vi "Configure.vi"(8 "error in":errorcluster, 11 "File Actor in":refnum<class "File Actor.lvclass">) -> (0 "error out":errorcluster, 3 "File Actor out":refnum<class "File Actor.lvclass">)   [LabVIEW 2016, in "File Library.lvlib" / "File Actor.lvclass"]
uses:
  File Actor.lvclass
  C:/Program Files (x86)/National Instruments/LabVIEW 2016/vi.lib/ActorFramework/Actor/Actor.lvclass
  C:/Program Files (x86)/National Instruments/LabVIEW 2016/vi.lib/MSR Consulting, LLC/General Reuse/SuperActor/SuperActor.lvclass
  <vilib>/MSR Consulting, LLC/General Reuse/Session APIs/File Access/Config Data/Config Data.lvclass
  Messages/To/Save/Change File Writing State MSG.lvclass
  C:/Program Files (x86)/National Instruments/LabVIEW 2016/vi.lib/ActorFramework/Message/Message.lvclass
  <vilib>/ActorFramework/Actor/Actor.lvclass/Actor.ctl
  <vilib>/ActorFramework/Message Enqueuer/Message Enqueuer.lvclass/Message Enqueuer.ctl
  File Actor.lvclass/File Actor.ctl
  <vilib>/MSR Consulting, LLC/General Reuse/SuperActor/SuperActor.lvclass/SuperActor.ctl
  <vilib>/MSR Consulting, LLC/General Reuse/Session APIs/File Access/Config Data/Config Data.lvclass/Config Data.ctl
  Messages/To/Save/Change File Writing State MSG.lvclass/Change File Writing State MSG.ctl
  Read Cfg Header.vi
  <vilib>/MSR Consulting, LLC/General Reuse/SuperActor/Read ID.vi
  <vilib>/MSR Consulting, LLC/General Reuse/SuperActor/Read Config Session.vi
  <vilib>/MSR Consulting, LLC/General Reuse/Session APIs/File Access/Config Data/Accessors/Read Ref.vi
  Messages/To/Save/Write Save_.vi
  <vilib>/ActorFramework/Message Enqueuer/Init from Existing Queue.vi
  <vilib>/Utility/config.llb/Read Key (String).vi
  <vilib>/Utility/config.llb/Read Key (Boolean).vi
  <vilib>/Utility/config.llb/Read Key (I32).vi
  <vilib>/ActorFramework/Message Priority Queue/Priority Enqueue.vi
  <vilib>/ActorFramework/Message Enqueuer/Message Enqueuer.lvclass
  <vilib>/MSR Consulting, LLC/General Reuse/Session APIs/_Session Fwk/Session - Root.lvclass
  <vilib>/Utility/config.llb/NI_LVConfig.lvlib
  <vilib>/ActorFramework/Actor/Actor.lvclass
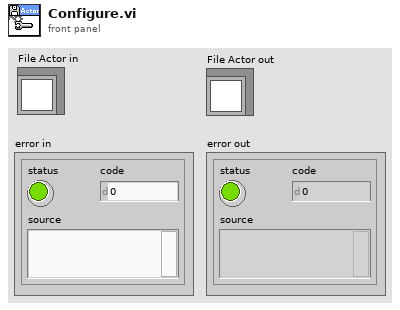
[diagram p1: front panel]
types:
  T1 = typedef "Session - Root.lvclass/Session Handle.ctl" = refnum<data-value>
  T2 = typedef "NI_LVConfig.lvlib/Config Data RefNum.ctl" = refnum<k1>
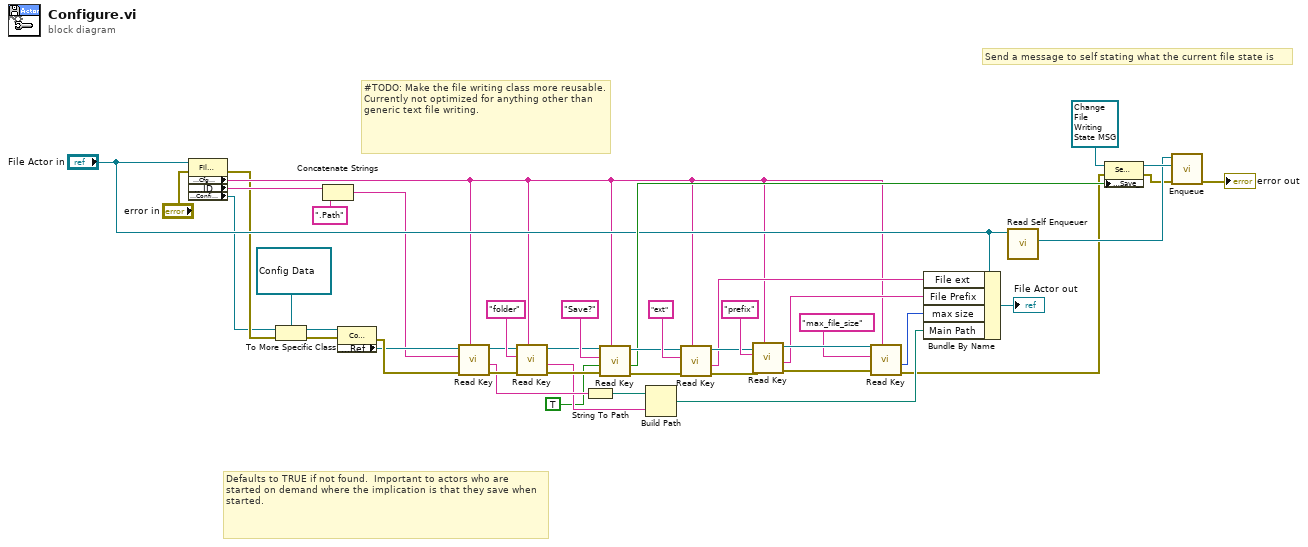
[diagram p0: block diagram]
diagram:
  # "Defaults to TRUE if not found.  Important to actors who are started on demand where the implication is that they save when started."
  # "Send a message to self stating what the current file state is"
  # "#TODO: Make the file writing class more reusable.  Currently not optimized for anything other than generic text file writing."
  n1 = property class="File Actor.lvclass"(reference="File Actor in", error in="error in") -> (error out=w3:errorcluster, "Accessors:Cfg Header"=w14:string, "Accessors:ID"=w11:string, "Accessors:Config Session"=w2:T1)  [unwired: 1 out]
  n2 = To More Specific Class(target class=refnum<data-value> refnum ("Config Session"), reference=w2, error in=w3) -> (specific class reference=w24:refnum<data-value>, error out=w25:errorcluster)
  n3 = Concatenate Strings(w11, ".Path" ("string")) -> (w12:string)
  n4 = property class="Config Data"(reference=w24, error in=w25) -> (error out=w43:errorcluster, "Accessors:Ref"=w26:T2)  [unwired: 1 out]
  n5 = call-poly <vilib>:"Read Key.vi"("section"=w14, "error in (no error)"=w43, "key"=w12, "refnum"=w26) -> ("error out"=w28:errorcluster, "value"=w22:string, "refnum out"=w27:T2)  [unwired: 4 in, 1 out]
  n6 = call-poly <vilib>:"Read Key.vi"("section"=w14, "error in (no error)"=w28, "key"="folder", "refnum"=w27) -> ("error out"=w31:errorcluster, "value"=w17:string, "refnum out"=w30:T2)  [unwired: 4 in, 1 out]
  n7 = String To Path(string=w22) -> (path=w16:path)
  n8 = call-poly <vilib>:"Read Key.vi"("section"=w14, "error in (no error)"=w31, "default value"=TRUE, "key"="Save?", "refnum"=w30) -> ("error out"=w34:errorcluster, "value"=w21:bool, "refnum out"=w33:T2)  [unwired: 3 in, 1 out]
  n9 = Build Path(base path=w16, name or relative path=w17) -> (appended path=w7:path)
  n10 = call-poly <vilib>:"Read Key.vi"("section"=w14, "error in (no error)"=w34, "key"="ext", "refnum"=w33) -> ("error out"=w38:errorcluster, "value"=w36:string, "refnum out"=w37:T2)  [unwired: 4 in, 1 out]
  n11 = call-poly <vilib>:"Read Key.vi"("section"=w14, "error in (no error)"=w38, "key"="prefix", "refnum"=w37) -> ("error out"=w42:errorcluster, "value"=w40:string, "refnum out"=w41:T2)  [unwired: 4 in, 1 out]
  n12 = call-poly <vilib>:"Read Key.vi"("section"=w14, "error in (no error)"=w42, "key"="max_file_size", "refnum"=w41) -> ("error out"=w6:errorcluster, "value"=w18:i32)  [unwired: 4 in, 2 out]
  n13 = Bundle By Name(cluster="File Actor in", "File ext"=w36, "File Prefix"=w40, "max size"=w18, "Main Path"=w7) -> (→"File Actor out":refnum<class "File Actor.lvclass">)
  n14 = call <vilib>:"Read Self Enqueuer.vi"("Actor"="File Actor in") -> ("Self Enqueuer"=w8:refnum<class "Message Enqueuer.lvclass">)  [unwired: 10 in]
  n15 = property class="Set File Save State"(reference=refnum<class "Change File Writing State MSG.lvclass"> refnum ("File Library.lvlib:Set File Save State"), error in=w6, "Accessors:Save_"=w21) -> (reference out=w9:refnum<class "Change File Writing State MSG.lvclass">, error out=w5:errorcluster)
  n16 = call <vilib>:"Enqueue.vi"("error in (no error)"=w5, "Message"=w9, "Message Enqueuer in"=w8) -> ("error out"=→"error out":errorcluster)  [unwired: 7 in, 1 out]
